vi "Crosstalk_sub.vi"(4 "% overtalk D-T1":u8, 5 "% overtalk D-T2":u8, 6 "% overtalk D-A":u8, 7 "MCS_bg_corr":dbl[][](array[numeric]) format="%.2f") -> (0 "Akzeptor":dbl[](array[numeric]) format="%.2f", 1 "Transmitter2":dbl[](array[numeric]) format="%.2f", 2 "Transmitter1":dbl[](array[numeric]) format="%.2f", 3 "MCS_crosstalk_corr":dbl[][](array[numeric]))   [LabVIEW 2009]
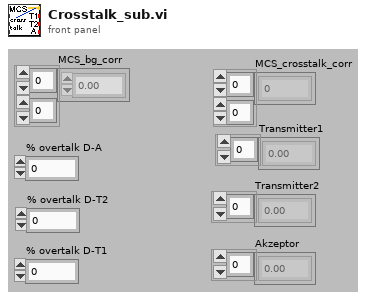
[diagram p1: front panel]
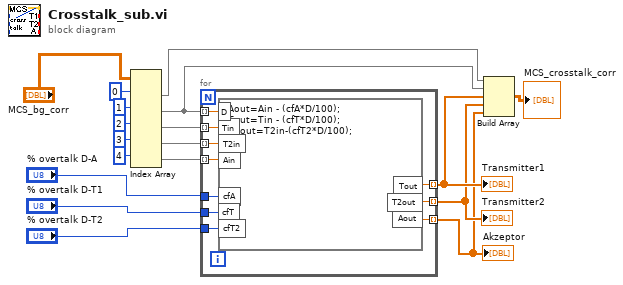
[diagram p0: block diagram]
diagram:
  n1 = Index Array(array="MCS_bg_corr", index (row) #1=0 ("index (row)"), index (row) #2=1 ("index (row)"), index (row) #3=2 ("index (row)"), index (row) #4=3 ("index (row)"), index (row) #5=4 ("index (row)")) -> (element #1=w1:dbl[], element #2=w7:dbl[], element #3=w14:dbl[], element #4=w15:dbl[], element #5=w18:dbl[])  [unwired: 5 in]
  n2 = for {
    tunnel: [w28] -> w4 mode=indexing
    tunnel: [w20] -> w5 mode=indexing
    tunnel: "% overtalk D-T2" -> [w27]
    tunnel: [w19] -> w6 mode=indexing
    tunnel: w7 -> [w26] mode=indexing
    tunnel: w14 -> [w25] mode=indexing
    tunnel: w15 -> [w24] mode=indexing
    tunnel: w18 -> [w23] mode=indexing
    tunnel: "% overtalk D-T1" -> [w22]
    tunnel: "% overtalk D-A" -> [w21]
    n3 = formula code="Aout=Ain - (cfA*D/100);\nTout=Tin - (cfT*D/100);\nT2out=T2in-(cfT2*D/100);"("Tin"=w25, "D"=w26, "cfA"=w21, "cfT"=w22, "Ain"=w23, "cfT2"=w27, "T2in"=w24) -> ("Aout"=w28:dbl, "Tout"=w19:dbl, "T2out"=w20:dbl)
  }
  "Transmitter1" <- w6
  "Akzeptor" <- w4
  "Transmitter2" <- w5
  n4 = Build Array(w1, w7, w6, w5, w4) -> (→"MCS_crosstalk_corr":dbl[][])
